vi "三维曲线.vi"() -> ()   [LabVIEW 2010]
uses:
  <vilib>/Platform/NI_3dgraph.lvlib
  <vilib>/Analysis/NI_AALBase.lvlib
panel:
  in  "三维曲线":refnum<k7>(container)
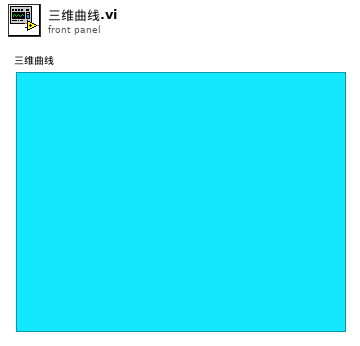
[diagram p1: front panel]
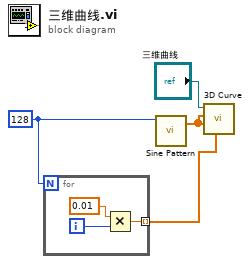
[diagram p0: block diagram]
diagram:
  w1 = 128
  n1 = for {
    N: w1 -> [_]
    tunnel: [w6] -> w2 mode=indexing
    i -> [w7]
    n2 = Multiply(x=0.01, y=w7) -> (x*y=w6:dbl)
  }
  n3 = call <vilib>:"Sine Pattern.vi"("samples"=w1) -> ("Sinusoidal Pattern"=w3:dbl[])  [unwired: 3 in, 1 out]
  n4 = call <vilib>:"3D Curve.vi"("z vector"=w2, "y vector"=w3, "x vector"=w3, "3D graph"="三维曲线") -> ()  [unwired: 6 in, 2 out]
